vi "StreamReceiveInstrument.vi"() -> ()   [LabVIEW 2018]
panel:
  in  "stop 2":bool
  out "error out":errorcluster
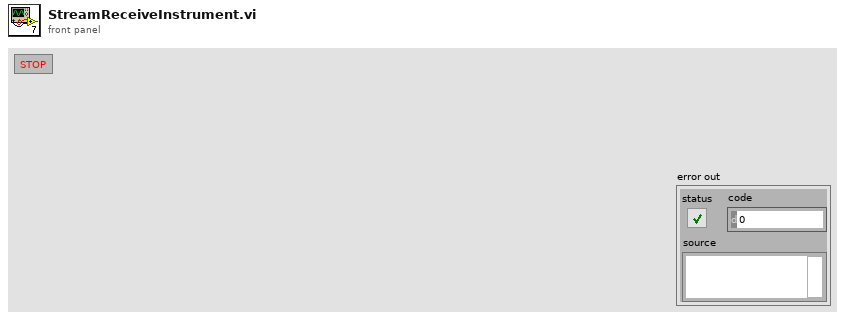
[diagram p1: front panel]
types:
  T1 = enum16{"Standard", "Buffered", "CRLF", "Immediate"}
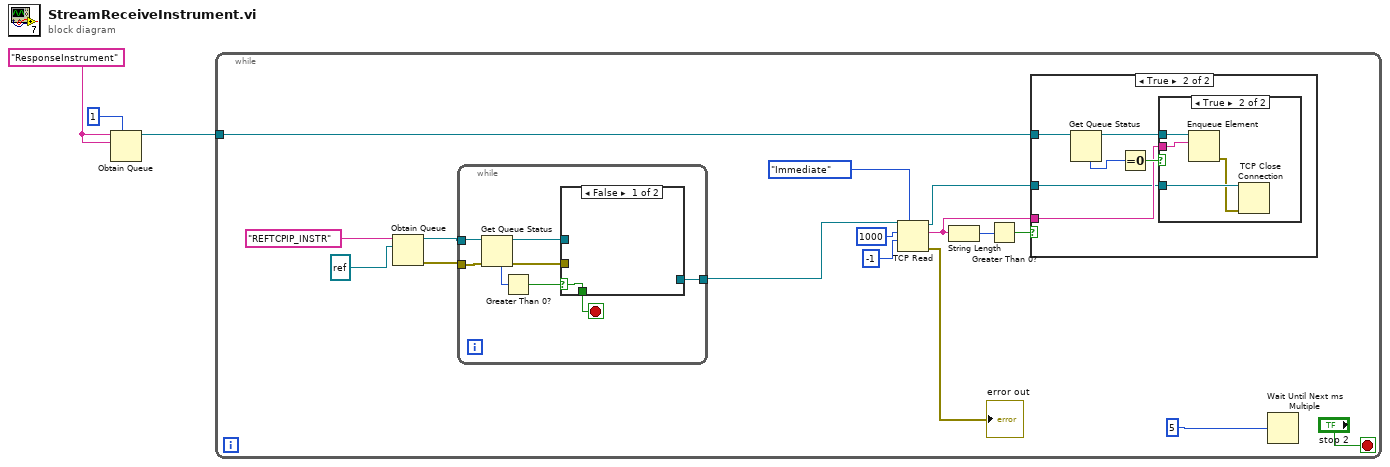
[diagram p0: block diagram]
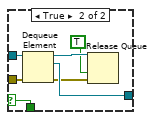
[diagram p2: hidden frame]
diagram:
  w3 = "ResponseInstrument"
  n1 = Obtain Queue(max queue size (-1, unlimited)=1, name (unnamed)=w3, element data type=w3) -> (queue out=w2:refnum<queue>)  [unwired: 2 in, 2 out]
  n2 = while {
    tunnel: w2 -> [w18]
    stop <- "stop 2" stop-if-true
    n3 = Obtain Queue(name (unnamed)="REFTCPIP_INSTR", element data type=refnum<k5> refnum ("connection ID out")) -> (queue out=w5:refnum<queue>, error out=w4:errorcluster)  [unwired: 3 in, 1 out]
    n4 = while {
      tunnel: [w22] -> w8
      tunnel: w5 -> [w21]
      tunnel: w4 -> [w20]
      stop <- w23 stop-if-true
      n5 = Get Queue Status(queue=w21, error in (no error)=w20) -> (queue out=w27:refnum<queue>, error out=w26:errorcluster, # elements in queue=w24:i32)  [unwired: 1 in, 5 out]
      n6 = Greater Than 0?(x=w24) -> (x > 0?=w25:bool)
      n7 = case shown="False" w25 {
        selector: w25 -> [w28 w33]
        tunnel: w27 -> [_ w35]
        tunnel: w26 -> [_ w34]
        tunnel: [w28 w33] -> w23
        tunnel: [_ w32] -> w22
        frame False {
        }
        frame True {
          n8 = Dequeue Element(queue=w35, error in (no error)=w34) -> (queue out=w31:refnum<queue>, element=w32:refnum<k5>, error out=w30:errorcluster)  [unwired: 1 in, 1 out]
          n9 = Release Queue(queue=w31, force destroy? (F)=TRUE, error in (no error)=w30) -> ()  [unwired: 3 out]
        }
      }
    }
    n10 = TCP Read(connection ID=w8, bytes to read=1000, 7:T1."Immediate" ("mode (standard)"), 9:-1 ("bytes to read")) -> (connection ID out=w9:refnum<k5>, data out=w14:string, error out=→"error out":errorcluster)  [unwired: 1 in]
    n11 = String Length(string=w14) -> (length=w16:i32)
    n12 = Greater Than 0?(x=w16) -> (x > 0?=w15:bool)
    n13 = case shown="True" w15 {
      tunnel: w18 -> [_ w39]
      tunnel: w14 -> [_ w37]
      tunnel: w9 -> [_ w36]
      frame False {
      }
      frame True {
        n14 = Get Queue Status(queue=w39) -> (queue out=w38:refnum<queue>, # elements in queue=w41:i32)  [unwired: 2 in, 6 out]
        n15 = Equal To 0?(x=w41) -> (x = 0?=w40:bool)
        n16 = case shown="True" w40 {
          tunnel: w38 -> [_ w45]
          tunnel: w37 -> [_ w44]
          tunnel: w36 -> [_ w43]
          frame False {
          }
          frame True {
            n17 = Enqueue Element(queue=w45, element=w44) -> (error out=w42:errorcluster)  [unwired: 2 in, 2 out]
            n18 = TCP Close Connection(connection ID=w43, error in (no error)=w42) -> ()  [unwired: 1 in, 2 out]
          }
        }
      }
    }
    n19 = Wait Until Next ms Multiple(millisecond multiple=u32 5) -> ()  [unwired: 1 out]
  }
